vi "all refs.vi"(1 "VI":refnum<vi>) -> (0 "all controls":refnum<vi>[](array[refnum]))   [LabVIEW 2012]
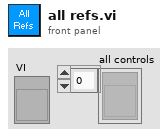
[diagram p1: front panel]
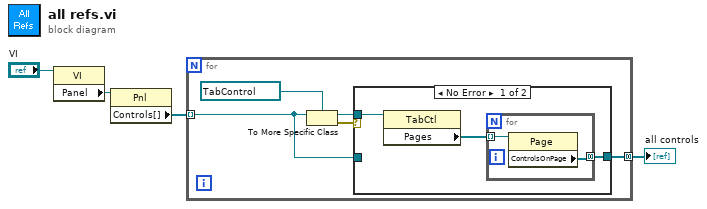
[diagram p0: block diagram]
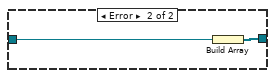
[diagram p2: hidden frame]
diagram:
  n1 = property class="VI"(reference="VI") -> ("Panel"=w4:refnum<vi>)  [unwired: 1 in, 2 out]
  n2 = property class="Pnl"(reference=w4) -> ("Controls[]"=w3:refnum<vi>[])  [unwired: 1 in, 2 out]
  n3 = for {
    tunnel: w3 -> [w6] mode=indexing
    tunnel: [w5] -> w1 mode=concatenating
    n4 = To More Specific Class(target class=refnum<vi> refnum ("reference"), reference=w6) -> (specific class reference=w8:refnum<vi>, error out=w7:errorcluster)  [unwired: 1 in]
    n5 = case shown="No Error" w7 {
      tunnel: w8 -> [w12 _]
      tunnel: [w10 w16] -> w5
      tunnel: w6 -> [_ w15]
      frame No Error {
        n6 = property on="Property Node" class="TabCtl"(reference=w12) -> ("Pages"=w11:refnum<vi>[])  [unwired: 1 in, 2 out]
        n7 = for {
          tunnel: w11 -> [w14] mode=indexing
          tunnel: [w13] -> w10 mode=concatenating
          n8 = property class="Page"(reference=w14) -> ("ControlsOnPage"=w13:refnum<vi>[])  [unwired: 1 in, 2 out]
        }
      }
      frame Error {
        n9 = Build Array(w15) -> (w16:refnum<vi>[])
      }
    }
  }
  "all controls" <- w1
